vi "RichToFlatnidaqmx_grpc_SetChanAttributeDoubleRequest.vi"(5 "OutputClusterType":T1, 11 "InputCluster":T4) -> (3 "OutputCluster":T1)   [LabVIEW 2021, in "NI_DAQmx_client.lvlib"]
uses:
  NI_DAQmx_client.lvlib
  nidaqmx_grpc_SetChanAttributeDoubleRequest.ctl
  nidevice_grpc_Session_session/nidevice_grpc_Session_session.lvclass
  nidaqmx_grpc_SetChanAttributeDoubleRequest_attribute_enum/nidaqmx_grpc_SetChanAttributeDoubleRequest_attribute_enum.lvclass
  nidevice_grpc_Session.ctl
  nidaqmx_grpc_SetChanAttributeDoubleRequest_Flat.ctl
  nidevice_grpc_Session_Flat.ctl
  nidaqmx_grpc_ChannelDoubleAttribute.ctl
  nidevice_grpc_Session_session/nidevice_grpc_Session_session.lvclass/nidevice_grpc_Session_session.ctl
  nidaqmx_grpc_SetChanAttributeDoubleRequest_attribute_enum/nidaqmx_grpc_SetChanAttributeDoubleRequest_attribute_enum.lvclass/nidaqmx_grpc_SetChanAttributeDoubleRequest_attribute_enum.ctl
  nidevice_grpc_Session_session/Getname.vi
  nidevice_grpc_Session_session/Getid.vi
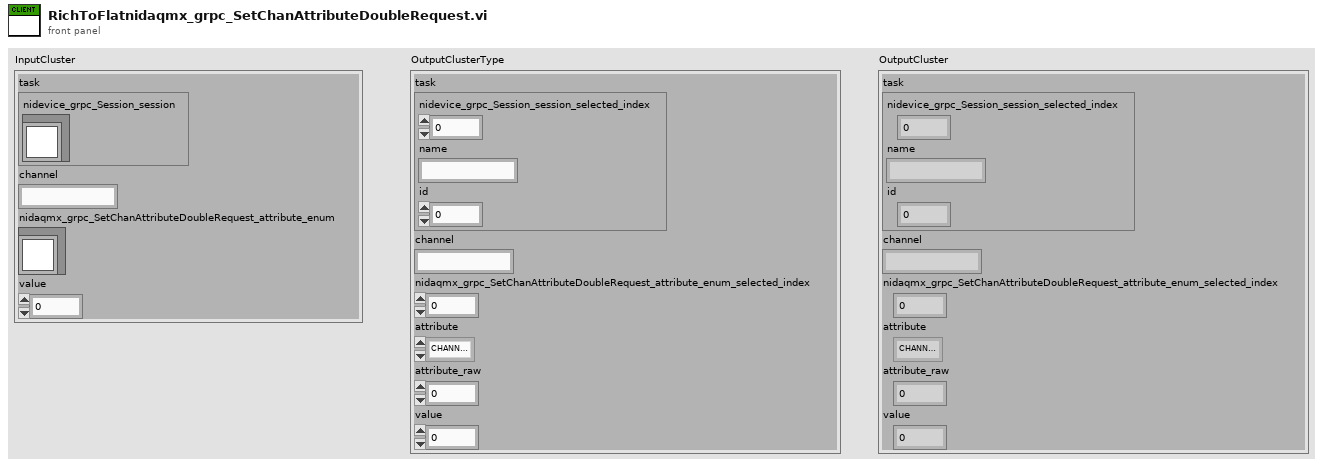
[diagram p1: front panel]
types:
  T1 = typedef "NI_DAQmx_client.lvlib/nidaqmx_grpc_SetChanAttributeDoubleRequest_Flat.ctl" = cluster{"task":T2, "channel":string, "nidaqmx_grpc_SetChanAttributeDoubleRequest_attribute_enum_selected_index":i32, "attribute":T3, "attribute_raw":i32, "value":dbl}
  T2 = typedef "NI_DAQmx_client.lvlib/nidevice_grpc_Session_Flat.ctl" = cluster{"nidevice_grpc_Session_session_selected_index":i32, "name":string, "id":u32}
  T3 = typedef "NI_DAQmx_client.lvlib/nidaqmx_grpc_ChannelDoubleAttribute.ctl" = enum32{"CHANNEL_DOUBLE_ATTRIBUTE_UNSPECIFIED", "CHANNEL_ATTRIBUTE_AI_IMPEDANCE", "CHANNEL_ATTRIBUTE_AI_AC_EXCIT_FREQ", "CHANNEL_ATTRIBUTE_AO_GAIN", "CHANNEL_ATTRIBUTE_AO_LOAD_IMPEDANCE", "CHANNEL_ATTRIBUTE_CI_FREQ_MEAS_TIME", "CHANNEL_ATTRIBUTE_CO_PULSE_FREQ_INITIAL_DELAY", "CHANNEL_ATTRIBUTE_AI_ACCEL_SENSITIVITY", "CHANNEL_ATTRIBUTE_AI_FREQ_HYST", "CHANNEL_ATTRIBUTE_AI_FREQ_THRESH_VOLTAGE", "CHANNEL_ATTRIBUTE_CI_ANG_ENCODER_INITIAL_ANGLE", "CHANNEL_ATTRIBUTE_CI_ENCODER_Z_INDEX_VAL", "CHANNEL_ATTRIBUTE_AI_RVDT_SENSITIVITY", "CHANNEL_ATTRIBUTE_CI_LIN_ENCODER_DIST_PER_PULSE", "CHANNEL_ATTRIBUTE_CI_LIN_ENCODER_INITIAL_POS", "CHANNEL_ATTRIBUTE_AI_LVDT_SENSITIVITY", "CHANNEL_ATTRIBUTE_AI_STRAIN_GAGE_GAGE_FACTOR", "CHANNEL_ATTRIBUTE_AI_STRAIN_GAGE_POISSON_RATIO", "CHANNEL_ATTRIBUTE_AI_RTD_A", "CHANNEL_ATTRIBUTE_AI_RTD_B", "CHANNEL_ATTRIBUTE_AI_RTD_C", "CHANNEL_ATTRIBUTE_AI_RTD_R0", "CHANNEL_ATTRIBUTE_AI_THRMCPL_CJC_VAL", "CHANNEL_ATTRIBUTE_AI_THRMSTR_R1", "CHANNEL_ATTRIBUTE_CO_PULSE_DUTY_CYC", "CHANNEL_ATTRIBUTE_CO_PULSE_FREQ", "CHANNEL_ATTRIBUTE_AO_MAX", "CHANNEL_ATTRIBUTE_AO_MIN", "CHANNEL_ATTRIBUTE_AO_OUTPUT_IMPEDANCE", "CHANNEL_ATTRIBUTE_AI_MICROPHONE_SENSITIVITY", "CHANNEL_ATTRIBUTE_AI_RESOLUTION", "CHANNEL_ATTRIBUTE_AI_MAX", "CHANNEL_ATTRIBUTE_AI_MIN", "CHANNEL_ATTRIBUTE_AI_BRIDGE_NOM_RESISTANCE", "CHANNEL_ATTRIBUTE_AI_BRIDGE_INITIAL_VOLTAGE", "CHANNEL_ATTRIBUTE_AI_LEAD_WIRE_RESISTANCE", "CHANNEL_ATTRIBUTE_AI_CURRENT_SHUNT_RESISTANCE", "CHANNEL_ATTRIBUTE_AI_EXCIT_VAL", "CHANNEL_ATTRIBUTE_AI_ATTEN", "CHANNEL_ATTRIBUTE_AI_LOWPASS_CUTOFF_FREQ", "CHANNEL_ATTRIBUTE_AI_HIGHPASS_CUTOFF_FREQ", "CHANNEL_ATTRIBUTE_AI_BANDPASS_CENTER_FREQ", "CHANNEL_ATTRIBUTE_AI_BANDPASS_WIDTH", "CHANNEL_ATTRIBUTE_AI_NOTCH_CENTER_FREQ", "CHANNEL_ATTRIBUTE_AI_NOTCH_WIDTH", "CHANNEL_ATTRIBUTE_AI_RNG_HIGH", "CHANNEL_ATTRIBUTE_AI_RNG_LOW", "CHANNEL_ATTRIBUTE_AI_GAIN", "CHANNEL_ATTRIBUTE_AO_RESOLUTION", "CHANNEL_ATTRIBUTE_AO_DAC_RNG_LOW", "CHANNEL_ATTRIBUTE_AO_DAC_RNG_HIGH", "CHANNEL_ATTRIBUTE_AO_DAC_REF_VAL", "CHANNEL_ATTRIBUTE_AI_EXCIT_ACTUAL_VAL", "CHANNEL_ATTRIBUTE_AI_LOWPASS_SWITCH_CAP_EXT_CLK_FREQ", "CHANNEL_ATTRIBUTE_CI_MAX", "CHANNEL_ATTRIBUTE_CI_MIN", "CHANNEL_ATTRIBUTE_CI_CTR_TIMEBASE_RATE", "CHANNEL_ATTRIBUTE_CO_PULSE_HIGH_TIME", "CHANNEL_ATTRIBUTE_CO_PULSE_LOW_TIME", "CHANNEL_ATTRIBUTE_CO_PULSE_TIME_INITIAL_DELAY", "CHANNEL_ATTRIBUTE_CO_CTR_TIMEBASE_RATE", "CHANNEL_ATTRIBUTE_AI_THRMSTR_A", "CHANNEL_ATTRIBUTE_AI_THRMSTR_C", "CHANNEL_ATTRIBUTE_AI_THRMSTR_B", "CHANNEL_ATTRIBUTE_CI_PERIOD_MEAS_TIME", "CHANNEL_ATTRIBUTE_AI_BRIDGE_SHUNT_CAL_GAIN_ADJUST", "CHANNEL_ATTRIBUTE_DI_DIG_FLTR_MIN_PULSE_WIDTH", "CHANNEL_ATTRIBUTE_CI_FREQ_DIG_FLTR_MIN_PULSE_WIDTH", "CHANNEL_ATTRIBUTE_CI_FREQ_DIG_FLTR_TIMEBASE_RATE", "CHANNEL_ATTRIBUTE_CI_PERIOD_DIG_FLTR_MIN_PULSE_WIDTH", "CHANNEL_ATTRIBUTE_CI_PERIOD_DIG_FLTR_TIMEBASE_RATE", "CHANNEL_ATTRIBUTE_CI_COUNT_EDGES_COUNT_DIR_DIG_FLTR_MIN_PULSE_WIDTH", "CHANNEL_ATTRIBUTE_CI_COUNT_EDGES_COUNT_DIR_DIG_FLTR_TIMEBASE_RATE", "CHANNEL_ATTRIBUTE_CI_COUNT_EDGES_DIG_FLTR_MIN_PULSE_WIDTH", "CHANNEL_ATTRIBUTE_CI_COUNT_EDGES_DIG_FLTR_TIMEBASE_RATE", "CHANNEL_ATTRIBUTE_CI_ENCODER_A_INPUT_DIG_FLTR_MIN_PULSE_WIDTH", "CHANNEL_ATTRIBUTE_CI_ENCODER_A_INPUT_DIG_FLTR_TIMEBASE_RATE", "CHANNEL_ATTRIBUTE_CI_ENCODER_B_INPUT_DIG_FLTR_MIN_PULSE_WIDTH", "CHANNEL_ATTRIBUTE_CI_ENCODER_B_INPUT_DIG_FLTR_TIMEBASE_RATE", "CHANNEL_ATTRIBUTE_CI_ENCODER_Z_INPUT_DIG_FLTR_MIN_PULSE_WIDTH", "CHANNEL_ATTRIBUTE_CI_ENCODER_Z_INPUT_DIG_FLTR_TIMEBASE_RATE", "CHANNEL_ATTRIBUTE_CI_PULSE_WIDTH_DIG_FLTR_MIN_PULSE_WIDTH", "CHANNEL_ATTRIBUTE_CI_PULSE_WIDTH_DIG_FLTR_TIMEBASE_RATE", "CHANNEL_ATTRIBUTE_CI_TWO_EDGE_SEP_FIRST_DIG_FLTR_MIN_PULSE_WIDTH", "CHANNEL_ATTRIBUTE_CI_TWO_EDGE_SEP_FIRST_DIG_FLTR_TIMEBASE_RATE", "CHANNEL_ATTRIBUTE_CI_TWO_EDGE_SEP_SECOND_DIG_FLTR_MIN_PULSE_WIDTH", "CHANNEL_ATTRIBUTE_CI_TWO_EDGE_SEP_SECOND_DIG_FLTR_TIMEBASE_RATE", "CHANNEL_ATTRIBUTE_CI_SEMI_PERIOD_DIG_FLTR_MIN_PULSE_WIDTH", "CHANNEL_ATTRIBUTE_CI_SEMI_PERIOD_DIG_FLTR_TIMEBASE_RATE", "CHANNEL_ATTRIBUTE_AI_SOUND_PRESSURE_MAX_SOUND_PRESSURE_LVL", "CHANNEL_ATTRIBUTE_AO_DAC_OFFSET_VAL", "CHANNEL_ATTRIBUTE_CI_CTR_TIMEBASE_DIG_FLTR_MIN_PULSE_WIDTH", "CHANNEL_ATTRIBUTE_CI_CTR_TIMEBASE_DIG_FLTR_TIMEBASE_RATE", "CHANNEL_ATTRIBUTE_CO_CTR_TIMEBASE_DIG_FLTR_MIN_PULSE_WIDTH", "CHANNEL_ATTRIBUTE_CO_CTR_TIMEBASE_DIG_FLTR_TIMEBASE_RATE", "CHANNEL_ATTRIBUTE_AI_VOLTAGE_DB_REF", "CHANNEL_ATTRIBUTE_AI_SOUND_PRESSURE_DB_REF", "CHANNEL_ATTRIBUTE_AI_ACCEL_DB_REF", "CHANNEL_ATTRIBUTE_AO_FUNC_GEN_FREQ", "CHANNEL_ATTRIBUTE_AO_FUNC_GEN_AMPLITUDE", "CHANNEL_ATTRIBUTE_AO_FUNC_GEN_OFFSET", "CHANNEL_ATTRIBUTE_AO_FUNC_GEN_SQUARE_DUTY_CYCLE", "CHANNEL_ATTRIBUTE_AO_VOLTAGE_CURRENT_LIMIT", "CHANNEL_ATTRIBUTE_AO_FUNC_GEN_FM_DEVIATION", "CHANNEL_ATTRIBUTE_DO_OVERCURRENT_LIMIT", "CHANNEL_ATTRIBUTE_DO_OVERCURRENT_REENABLE_PERIOD", "CHANNEL_ATTRIBUTE_AI_PROBE_ATTEN", "CHANNEL_ATTRIBUTE_AI_DC_OFFSET", "CHANNEL_ATTRIBUTE_AI_EDDY_CURRENT_PROX_PROBE_SENSITIVITY", "CHANNEL_ATTRIBUTE_DI_DIG_FLTR_TIMEBASE_RATE", "CHANNEL_ATTRIBUTE_CI_PULSE_FREQ_DIG_FLTR_MIN_PULSE_WIDTH", "CHANNEL_ATTRIBUTE_CI_PULSE_FREQ_DIG_FLTR_TIMEBASE_RATE", "CHANNEL_ATTRIBUTE_CI_PULSE_TIME_DIG_FLTR_MIN_PULSE_WIDTH", "CHANNEL_ATTRIBUTE_CI_PULSE_TIME_DIG_FLTR_TIMEBASE_RATE", "CHANNEL_ATTRIBUTE_CI_PULSE_TICKS_DIG_FLTR_MIN_PULSE_WIDTH", "CHANNEL_ATTRIBUTE_CI_PULSE_TICKS_DIG_FLTR_TIMEBASE_RATE", "CHANNEL_ATTRIBUTE_AI_BRIDGE_SHUNT_CAL_SHUNT_CAL_A_RESISTANCE", "CHANNEL_ATTRIBUTE_AI_BRIDGE_SHUNT_CAL_SHUNT_CAL_A_ACTUAL_RESISTANCE", "CHANNEL_ATTRIBUTE_AI_BRIDGE_SHUNT_CAL_SHUNT_CAL_B_RESISTANCE", "CHANNEL_ATTRIBUTE_AI_BRIDGE_SHUNT_CAL_SHUNT_CAL_B_ACTUAL_RESISTANCE", "CHANNEL_ATTRIBUTE_AI_FORCE_IEPE_SENSOR_SENSITIVITY", "CHANNEL_ATTRIBUTE_AI_BRIDGE_INITIAL_RATIO", "CHANNEL_ATTRIBUTE_AI_BRIDGE_TWO_POINT_LIN_FIRST_ELECTRICAL_VAL", "CHANNEL_ATTRIBUTE_AI_BRIDGE_TWO_POINT_LIN_FIRST_PHYSICAL_VAL", "CHANNEL_ATTRIBUTE_AI_BRIDGE_TWO_POINT_LIN_SECOND_ELECTRICAL_VAL", "CHANNEL_ATTRIBUTE_AI_BRIDGE_TWO_POINT_LIN_SECOND_PHYSICAL_VAL", "CHANNEL_ATTRIBUTE_CI_COUNT_EDGES_COUNT_RESET_DIG_FLTR_MIN_PULSE_WIDTH", "CHANNEL_ATTRIBUTE_CI_COUNT_EDGES_COUNT_RESET_DIG_FLTR_TIMEBASE_RATE", "CHANNEL_ATTRIBUTE_AI_THRMCPL_LEAD_OFFSET_VOLTAGE", "CHANNEL_ATTRIBUTE_AI_FILTER_DELAY", "CHANNEL_ATTRIBUTE_AI_VELOCITY_IEPE_SENSOR_DB_REF", "CHANNEL_ATTRIBUTE_AI_VELOCITY_IEPE_SENSOR_SENSITIVITY", "CHANNEL_ATTRIBUTE_AI_ROSETTE_STRAIN_GAGE_ORIENTATION", "CHANNEL_ATTRIBUTE_AO_FILTER_DELAY_ADJUSTMENT", "CHANNEL_ATTRIBUTE_AI_FILTER_DELAY_ADJUSTMENT", "CHANNEL_ATTRIBUTE_AO_FILTER_DELAY", "CHANNEL_ATTRIBUTE_CI_DUTY_CYCLE_DIG_FLTR_MIN_PULSE_WIDTH", "CHANNEL_ATTRIBUTE_CI_DUTY_CYCLE_DIG_FLTR_TIMEBASE_RATE", "CHANNEL_ATTRIBUTE_CI_MAX_MEAS_PERIOD", "CHANNEL_ATTRIBUTE_CI_THRESH_VOLTAGE", "CHANNEL_ATTRIBUTE_AI_DIG_FLTR_LOWPASS_CUTOFF_FREQ", "CHANNEL_ATTRIBUTE_AI_DIG_FLTR_HIGHPASS_CUTOFF_FREQ", "CHANNEL_ATTRIBUTE_AI_DIG_FLTR_BANDPASS_CENTER_FREQ", "CHANNEL_ATTRIBUTE_AI_DIG_FLTR_BANDPASS_WIDTH", "CHANNEL_ATTRIBUTE_AI_DIG_FLTR_NOTCH_CENTER_FREQ", "CHANNEL_ATTRIBUTE_AI_DIG_FLTR_NOTCH_WIDTH", "CHANNEL_ATTRIBUTE_CI_VELOCITY_LIN_ENCODER_DIST_PER_PULSE", "CHANNEL_ATTRIBUTE_CI_VELOCITY_ENCODER_A_INPUT_DIG_FLTR_MIN_PULSE_WIDTH", "CHANNEL_ATTRIBUTE_CI_VELOCITY_ENCODER_A_INPUT_DIG_FLTR_TIMEBASE_RATE", "CHANNEL_ATTRIBUTE_CI_VELOCITY_ENCODER_B_INPUT_DIG_FLTR_MIN_PULSE_WIDTH", "CHANNEL_ATTRIBUTE_CI_VELOCITY_ENCODER_B_INPUT_DIG_FLTR_TIMEBASE_RATE", "CHANNEL_ATTRIBUTE_CI_VELOCITY_MEAS_TIME", "CHANNEL_ATTRIBUTE_CI_COUNT_EDGES_GATE_DIG_FLTR_MIN_PULSE_WIDTH", "CHANNEL_ATTRIBUTE_CI_COUNT_EDGES_GATE_DIG_FLTR_TIMEBASE_RATE", "CHANNEL_ATTRIBUTE_AI_ACCEL_CHARGE_SENSITIVITY", "CHANNEL_ATTRIBUTE_AI_ACCEL_4_WIRE_DC_VOLTAGE_SENSITIVITY", "CHANNEL_ATTRIBUTE_AI_DATA_XFER_MAX_RATE", "CHANNEL_ATTRIBUTE_AI_SENSOR_POWER_VOLTAGE", "CHANNEL_ATTRIBUTE_AI_FILTER_FREQ", "CHANNEL_ATTRIBUTE_AI_INPUT_LIMITS_FAULT_DETECT_UPPER_LIMIT", "CHANNEL_ATTRIBUTE_AI_INPUT_LIMITS_FAULT_DETECT_LOWER_LIMIT", "CHANNEL_ATTRIBUTE_CI_FREQ_THRESH_VOLTAGE", "CHANNEL_ATTRIBUTE_CI_FREQ_HYST", "CHANNEL_ATTRIBUTE_CI_PERIOD_THRESH_VOLTAGE", "CHANNEL_ATTRIBUTE_CI_PERIOD_HYST", "CHANNEL_ATTRIBUTE_CI_COUNT_EDGES_THRESH_VOLTAGE", "CHANNEL_ATTRIBUTE_CI_COUNT_EDGES_HYST", "CHANNEL_ATTRIBUTE_CI_COUNT_EDGES_COUNT_DIR_THRESH_VOLTAGE", "CHANNEL_ATTRIBUTE_CI_COUNT_EDGES_COUNT_DIR_HYST", "CHANNEL_ATTRIBUTE_CI_COUNT_EDGES_COUNT_RESET_THRESH_VOLTAGE", "CHANNEL_ATTRIBUTE_CI_COUNT_EDGES_COUNT_RESET_HYST", "CHANNEL_ATTRIBUTE_CI_COUNT_EDGES_GATE_THRESH_VOLTAGE", "CHANNEL_ATTRIBUTE_CI_COUNT_EDGES_GATE_HYST", "CHANNEL_ATTRIBUTE_CI_FILTER_FREQ", "CHANNEL_ATTRIBUTE_CI_FILTER_DELAY", "CHANNEL_ATTRIBUTE_AO_FUNC_GEN_START_PHASE", "CHANNEL_ATTRIBUTE_AO_COMMON_MODE_OFFSET", "CHANNEL_ATTRIBUTE_PWR_VOLTAGE_SETPOINT", "CHANNEL_ATTRIBUTE_PWR_CURRENT_SETPOINT"}
  T4 = typedef "NI_DAQmx_client.lvlib/nidaqmx_grpc_SetChanAttributeDoubleRequest.ctl" = cluster{"task":T5, "channel":string, "nidaqmx_grpc_SetChanAttributeDoubleRequest_attribute_enum":refnum<class "nidaqmx_grpc_SetChanAttributeDoubleRequest_attribute_enum.lvclass">, "value":dbl}
  T5 = typedef "NI_DAQmx_client.lvlib/nidevice_grpc_Session.ctl" = cluster{"nidevice_grpc_Session_session":refnum<class "nidevice_grpc_Session_session.lvclass">}
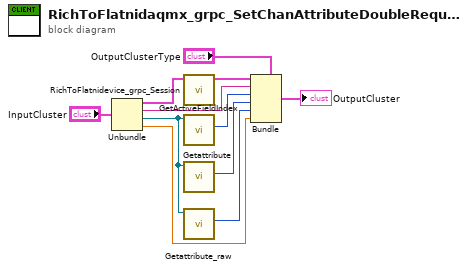
[diagram p0: block diagram]
diagram:
  n1 = Unbundle "Unbundle"("InputCluster") -> ("task"=w8:T5, "channel"=w6:string, "nidaqmx_grpc_SetChanAttributeDoubleRequest_attribute_enum"=w5:refnum<class "nidaqmx_grpc_SetChanAttributeDoubleRequest_attribute_enum.lvclass">, "value"=w1:dbl)
  n2 = call "RichToFlatnidevice_grpc_Session.vi"("InputCluster"=w8) -> ("OutputCluster"=w7:T2)  [unwired: 10 in]
  n3 = call "GetActiveFieldIndex.vi"("OneOfTemplate in"=w5) -> ("Active Field Index"=w4:i32)  [unwired: 8 in, 2 out]
  n4 = call "Getattribute.vi"("OneOfTemplate in"=w5) -> ("Get_Val"=w3:T3)  [unwired: 8 in, 2 out]
  n5 = call "Getattribute_raw.vi"("OneOfTemplate in"=w5) -> ("Get_Val"=w2:i32)  [unwired: 8 in, 2 out]
  n6 = Bundle "Bundle"(cluster="OutputClusterType", "task"=w7, "channel"=w6, "nidaqmx_grpc_SetChanAttributeDoubleRequest_attribute_enum_selected_index"=w4, "attribute"=w3, "attribute_raw"=w2, "value"=w1) -> (→"OutputCluster":T1)
